vi "filter_1pole.vi"(1 "beta":i32, 2 "IN":i32) -> (0 "OUT":i32)   [LabVIEW 2009]
doc: "Single pole filter. I32 filtered to I32. beta = exp(-1/d), where there are d samples per time constant. beta is I32."
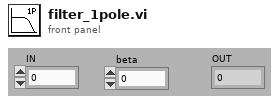
[diagram p1: front panel]
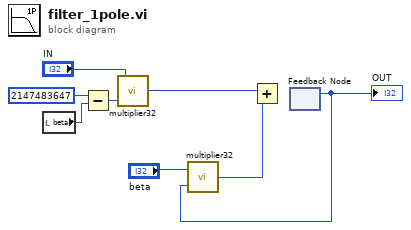
[diagram p0: block diagram]
diagram:
  n1 = local read "beta"() -> (w8:i32)
  n2 = Subtract(x=2147483647, y=w8) -> (x-y=w5:i32)
  n3 = call "multiplier32.vi"("Y"=w5, "X"="IN") -> ("XY"=w6:i32)
  n4 = feedback #1() -> (w3:i32)  [unwired: 1 in]
  "OUT" <- w3
  n5 = call "multiplier32.vi"("Y"=w3, "X"="beta") -> ("XY"=w1:i32)
  n6 = Add(x=w6, y=w1) -> (x+y=w7:i32)
